vi "Start Application.vi"(8 "error in (no error)":errorcluster, 11 "Application in":refnum<class "Application.lvclass">) -> (0 "error out":errorcluster, 3 "Application out":refnum<class "Application.lvclass">)   [LabVIEW 2017, in "Application.lvlib" / "Application.lvclass"]
doc: "Performs all start up methods for an Application Class."
uses:
  Application.lvclass
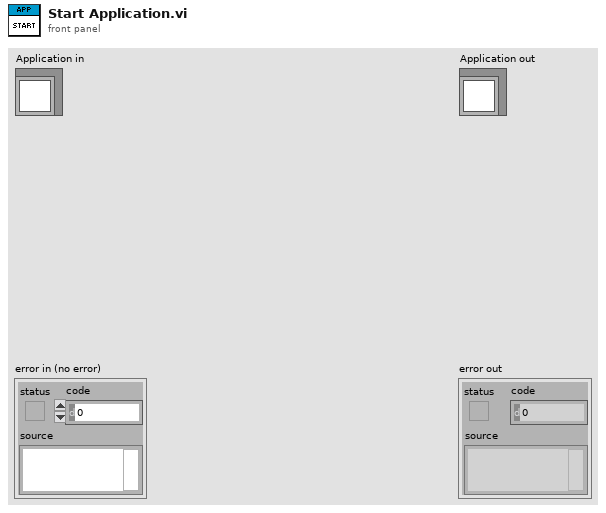
[diagram p1: front panel]
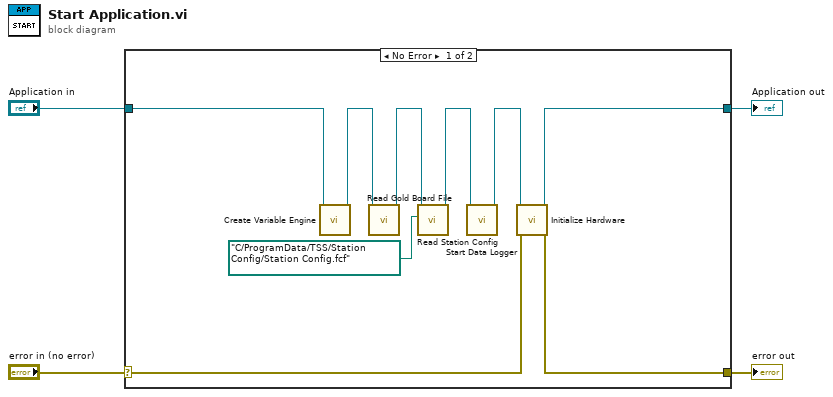
[diagram p0: block diagram]
diagram:
  n1 = case shown="No Error" "error in (no error)" {
    selector: "error in (no error)" -> [w10 w15]
    tunnel: [w12 w15] -> w3
    tunnel: [w13 w14] -> w1
    tunnel: "Application in" -> [w8 w14]
    frame No Error {
      n2 = call "Create Variable Engine.vi"("Application in"=w8) -> ("Application out"=w7:refnum<class "Application.lvclass">)  [unwired: 9 in, 1 out]
      n3 = call "Read Gold Board File.vi"("Application in"=w7) -> ("Application out"=w9:refnum<class "Application.lvclass">)  [unwired: 10 in]
      n4 = call "Read Station Config.vi"("Path to Config Folder"=path "C:/ProgramData/TSS/Station Config/Station Config.fcf", "Application in"=w9) -> ("Application out"=w6:refnum<class "Application.lvclass">)  [unwired: 9 in]
      n5 = call "Start Data Logger.vi"("Application in"=w6) -> ("Application out"=w11:refnum<class "Application.lvclass">)  [unwired: 10 in]
      n6 = call-dynamic "Initialize Hardware.vi"("error in (no error)"=w10, "Application in"=w11) -> ("error out"=w12:errorcluster, "Application out"=w13:refnum<class "Application.lvclass">)  [unwired: 8 in]
    }
    frame Error {
    }
  }
  "error out" <- w3
  "Application out" <- w1
